vi "NI9485.vi"() -> ()   [LabVIEW 2019]
panel:
  out "CH 1 ON":bool
  in  "Control CH 1":bool
  out "CH 0 ON":bool
  in  "Control CH 0":bool
  # "NI 9485 Control"
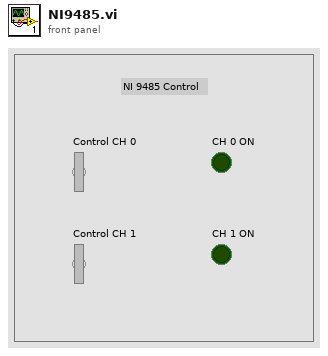
[diagram p1: front panel]
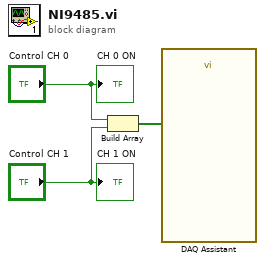
[diagram p0: block diagram]
diagram:
  n1 = Build Array("Control CH 0", "Control CH 1") -> (w1:bool[])
  n2 = call "DAQ Assistant"("data"=w1) -> ()  [unwired: 17 in, 2 out]
  "CH 0 ON" <- "Control CH 0"
  "CH 1 ON" <- "Control CH 1"
